vi "Target Address.vi"(6 "Addr. Mode":refnum<data-value>, 8 "error in (no error)":errorcluster, 11 "Low Speed in":refnum<class "Low Speed.lvclass">) -> (0 "error out":errorcluster, 3 "Low Speed out":refnum<class "Low Speed.lvclass">)   [LabVIEW 2020, in "Low Speed.lvclass"]
uses:
  Low Speed.lvclass
  C:/Users/kaiser.asan/OneDrive - SolitonTechnologies/LabVIEW/29.SDLC - I2C Driver/I2C Module/I2C Controller Module/Class/Transmission Mode/Parent/TX Speed.lvclass
  Addressing Mode/Parent/Addressing Mode.lvclass
  Parent/TX Speed.lvclass
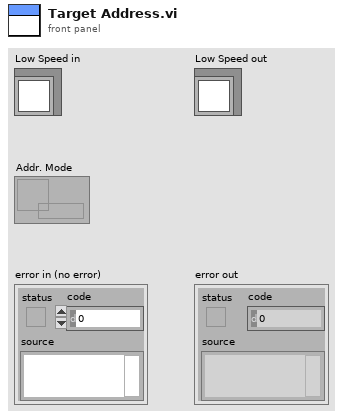
[diagram p1: front panel]
types:
  T1 = typedef "I2C Controller Lib.lvlib/Timing Parameters Cluster.ctl" = cluster{"f_SCL(KHz)":u32, "t_HIGH (ns)":u32, "t_LOW (ns)":u32, "t_SU;STA (ns)":u32, "t_HD;STA (ns)":u32, "t_SU;DAT (ns)":u32, "t_HD;DAT (ns)":u32, "t_SU;STO (ns)":u32, "t_BUF (ns)":u32}
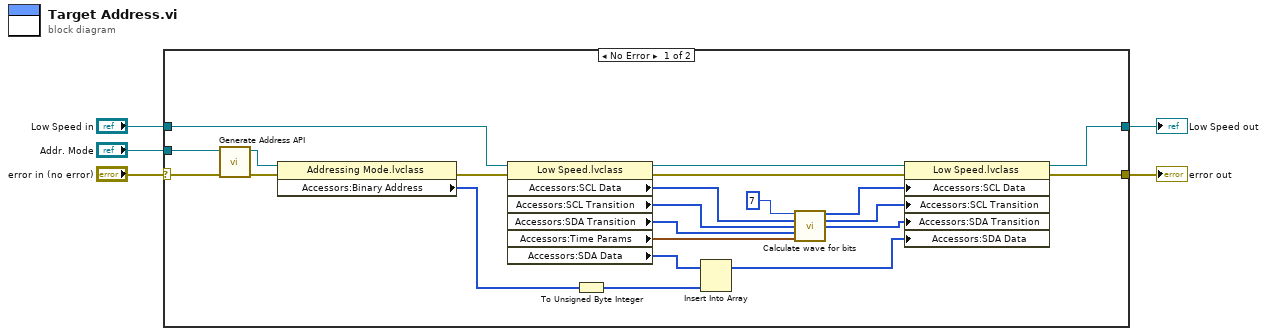
[diagram p0: block diagram]
diagram:
  n1 = case shown="No Error" "error in (no error)" {
    selector: "error in (no error)" -> [w26 w29]
    tunnel: [w19 w29] -> w5
    tunnel: [w18 w28] -> w4
    tunnel: "Low Speed in" -> [w22 w28]
    tunnel: "Addr. Mode" -> [w27 _]
    frame No Error {
      n2 = call "Generate Address API.vi"("error in (no error)"=w26, "DVR IN"=w27) -> ("error out"=w25:errorcluster, "DVR OUT"=w23:refnum<data-value>)  [unwired: 8 in]
      n3 = property class="Addressing Mode.lvclass"(reference=w23, error in=w25) -> (error out=w24:errorcluster, "Accessors:Binary Address"=w21:i16[])  [unwired: 1 out]
      n4 = property class="Low Speed.lvclass"(reference=w22, error in=w24) -> (reference out=w15:refnum<class "Low Speed.lvclass">, error out=w14:errorcluster, "Accessors:SCL Data"=w12:u8[], "Accessors:SCL Transition"=w11:u32[], "Accessors:SDA Transition"=w10:u32[], "Accessors:Time Params"=w9:T1, "Accessors:SDA Data"=w20:u8[])
      n5 = To Unsigned Byte Integer(number=w21) -> (unsigned 8bit integer=w16:u8[])
      n6 = Insert Into Array(array=w20, new element=w16) -> (w17:u8[])  [unwired: 1 in]
      n7 = call "Calculate wave for bits.vi"("No. Of Bits"=7, "SCL DATA IN"=w12, "SCL Transitions In"=w11, "SDA Transitions In"=w10, "Time Params"=w9) -> ("SCL DATA OUT"=w8:u8[], "SCL Transitions Out"=w7:u32[], "SDA Transitions Out"=w6:u32[])  [unwired: 8 in]
      n8 = property class="Low Speed.lvclass"(reference=w15, error in=w14, "Accessors:SCL Data"=w8, "Accessors:SCL Transition"=w7, "Accessors:SDA Transition"=w6, "Accessors:SDA Data"=w17) -> (reference out=w18:refnum<class "Low Speed.lvclass">, error out=w19:errorcluster)
    }
    frame Error {
    }
  }
  "error out" <- w5
  "Low Speed out" <- w4
